vi "Toggle Ancestors.vi"(8 "error in (no error)":errorcluster, 10 "Tag":string, 11 "TreeHier in":refnum<class "TreeSelectionHierarchal.lvclass">) -> (0 "error out":errorcluster, 3 "TreeHier out":refnum<class "TreeSelectionHierarchal.lvclass">)   [LabVIEW 2015, in "TreeSelectionHierarchal.lvclass"]
doc: "<b> </b> <b> </b>\n©2016 Q Software Innovations, LLC (QSI)\nwritten by Quentin Alldredge\nproduced in LabVIEW 2015\n\nsupport@qsoftwareinnovations.com\nwww.qsoftwareinnovations.com\n\nAll rights reserved.\n\nRedistribution and use in source and binary forms, with or without modification, are permitted provided that the following conditions are met:\n\n * Redistributions of source code must retain the above copyright notice, this list of conditions and the following disclaimer.\n * Redistributions in binary form must reproduce the above copyright notice, this list of conditions and the following disclaimer in the documentation and/or other materials provided with the distribution.\n * Neither the name of Q Software Innovations, LLC. nor the names of its contributors may be used to endorse or promote products derived from this software without specific prior written permission.\n\nTHIS SOFTWARE IS PROVIDED BY THE COPYRIGHT HOLDERS AND CONTRIBUTORS \"AS IS\" AND ANY EXPRESS OR IMPLIED WARRANTIES, INCLUDING, BUT NOT LIMITED TO, THE IMPLIED WARRANTIES OF MERCHANTABILITY AND FITNESS FOR A PARTICULAR PURPOSE ARE DISCLAIMED. IN NO EVENT SHALL THE COPYRIGHT OWNER OR CONTRIBUTORS BE LIABLE FOR ANY DIRECT, INDIRECT, INCIDENTAL, SPECIAL, EXEMPLARY, OR CONSEQUENTIAL DAMAGES (INCLUDING, BUT NOT LIMITED TO, PROCUREMENT OF SUBSTITUTE GOODS OR SERVICES; LOSS OF USE, DATA, OR PROFITS; OR BUSINESS INTERRUPTION) HOWEVER CAUSED AND ON ANY THEORY OF LIABILITY, WHETHER IN CONTRACT, STRICT LIABILITY, OR TORT (INCLUDING NEGLIGENCE OR OTHERWISE) ARISING IN ANY WAY OUT OF THE USE OF THIS SOFTWARE, EVEN IF ADVISED OF THE POSSIBILITY OF SUCH DAMAGE."
uses:
  TreeSelectionHierarchal.lvclass
  TreeSelectionHierarchal.lvclass/TreeSelectionHierarchal.ctl
  TreeControl/TreeControl.lvclass
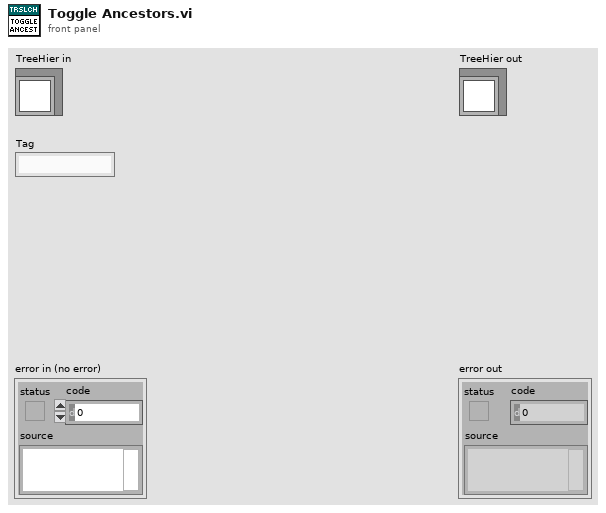
[diagram p1: front panel]
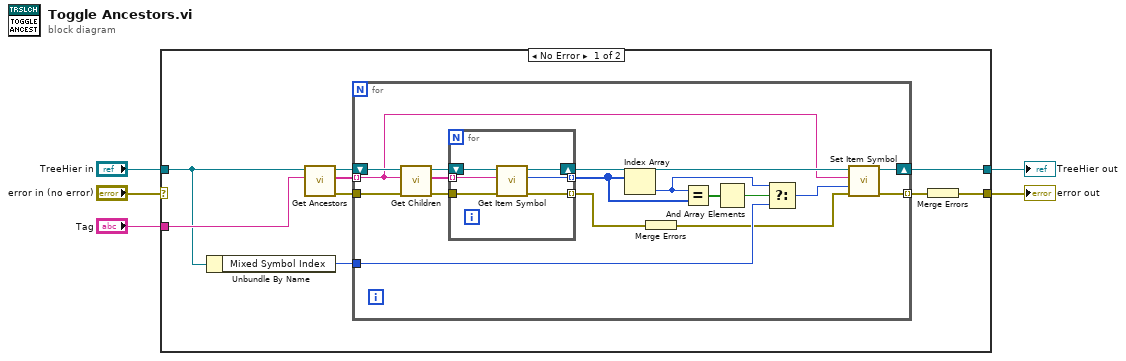
[diagram p0: block diagram]
diagram:
  n1 = case shown="No Error" "error in (no error)" {
    selector: "error in (no error)" -> [_ w39]
    tunnel: [w6 w39] -> w4
    tunnel: [w12 w38] -> w2
    tunnel: "TreeHier in" -> [w9 w38]
    tunnel: "Tag" -> [w14 _]
    frame No Error {
      n2 = Unbundle By Name(w9) -> ("Mixed Symbol Index"=w8:i32)
      n3 = call "Get Ancestors.vi"("Tag"=w14, "Tree in"=w9) -> ("error out"=w10:errorcluster, "Ancestors"=w11:string[], "Tree out"=w13:refnum<class "TreeSelectionHierarchal.lvclass">)  [unwired: 7 in]
      n4 = for {
        shift-right: [w23] -> w12
        shift-left: w13 -> [w31]
        tunnel: w11 -> [w22] mode=indexing
        tunnel: w10 -> [w29]
        tunnel: w8 -> [w20]
        tunnel: [w15] -> w7 mode=indexing
        n5 = call "Get Children.vi"("error in (no error)"=w29, "Tag"=w22, "Tree in"=w31) -> ("error out"=w18:errorcluster, "ChildrenTags[]"=w28:string[], "Tree out"=w30:refnum<class "TreeSelectionHierarchal.lvclass">)  [unwired: 6 in]
        n6 = for {
          shift-right: [w37] -> w24
          shift-left: w30 -> [w36]
          tunnel: w28 -> [w35] mode=indexing
          tunnel: [w34] -> w27 mode=indexing
          tunnel: w18 -> [w33]
          tunnel: [w32] -> w17 mode=indexing
          n7 = call "Get Item Symbol.vi"("error in (no error)"=w33, "Tag"=w35, "Tree in"=w36) -> ("error out"=w32:errorcluster, "Symbol Index"=w34:i32, "Tree out"=w37:refnum<class "TreeSelectionHierarchal.lvclass">)  [unwired: 6 in]
        }
        n8 = Index Array(array=w27) -> (element=w21:i32)  [unwired: 1 in]
        n9 = Merge Errors(w17) -> (w16:errorcluster)
        n10 = Equal?(x=w21, y=w27) -> (x = y?=w26:bool[])
        n11 = And Array Elements(Boolean array=w26) -> (logical AND=w25:bool)
        n12 = Select(t=w21, s=w25, f=w20) -> (s? t:f=w19:i32)
        n13 = call "Set Item Symbol.vi"("error in (no error)"=w16, "Symbol Index"=w19, "Tag"=w22, "Tree in"=w24) -> ("error out"=w15:errorcluster, "Tree (dup)"=w23:refnum<class "TreeSelectionHierarchal.lvclass">)  [unwired: 6 in]
      }
      n14 = Merge Errors(w7) -> (w6:errorcluster)
    }
    frame Error {
    }
  }
  "error out" <- w4
  "TreeHier out" <- w2
